vi "8.11.-Momentos Invariantes de Hu - Reconocimiento Patrones.vi"(7 "Normalización":bool, 9 "UMBRAL":dbl(knob) scale=0.0..255.0, 10 "CAPA DE COLOR":T1(ring), 11 "RUTA DE IMAGEN":path) -> (2 "Momentos Invariantes de Hu":dbl[](array[numeric]), 3 "IMAGEN BINARIZADA":picture)   [LabVIEW 2020]
panel:
  in  "Filtro Invertido":bool
  # "Visión Artificial - Momentos Invariantes de Hu\nDiego Cervantes Rodríguez\ndicer0.com"
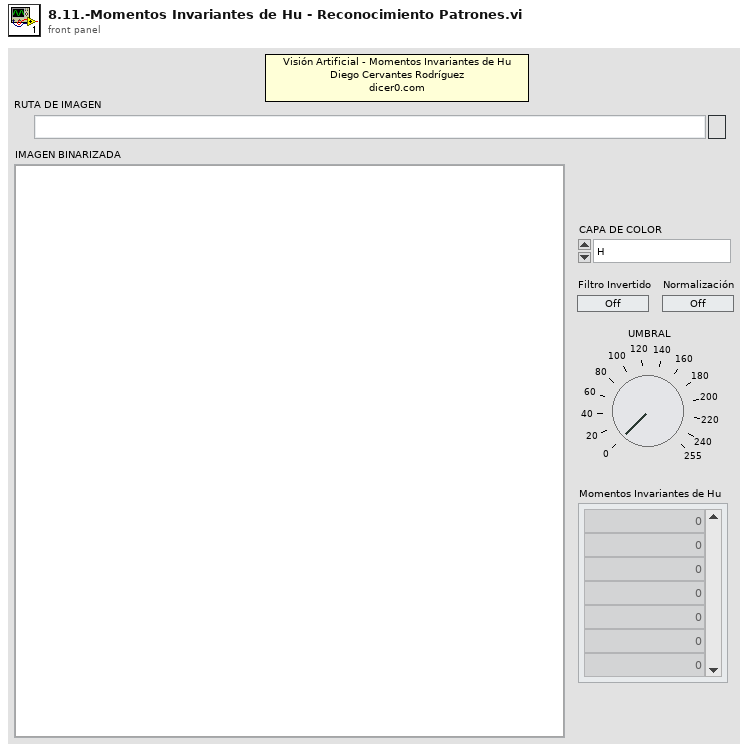
[diagram p1: front panel]
types:
  T1 = enum16{"H", "S", "V", "C", "M", "Y", "R", "G", "B", "RGB2GRAY MATLAB"}
  T2 = typedef "imagedata.ctl" = cluster{"image type":i32, "image depth":i32, "image":u8[], "mask":u8[], "colors":u32[], "Rectangle":cluster{"left":i16, "top":i16, "right":i16, "bottom":i16}}
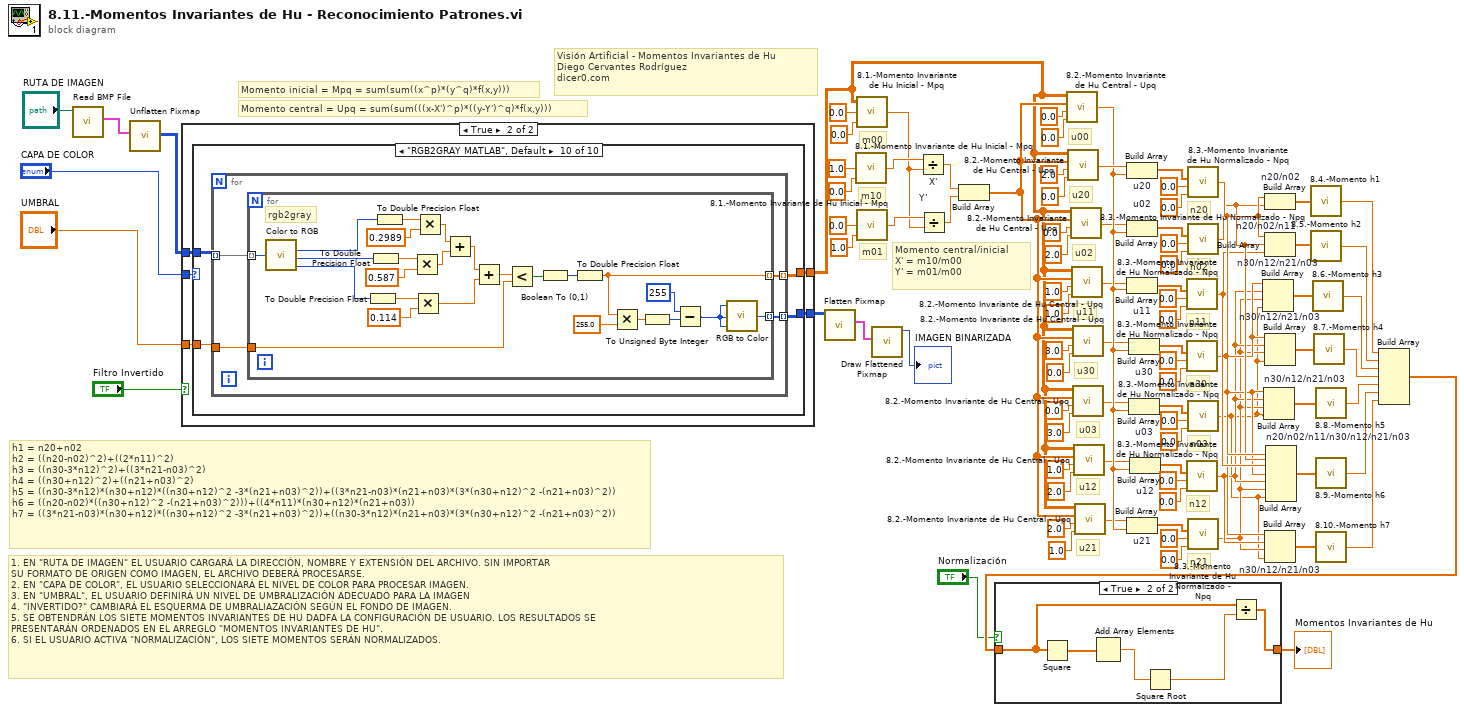
[diagram p0: block diagram]
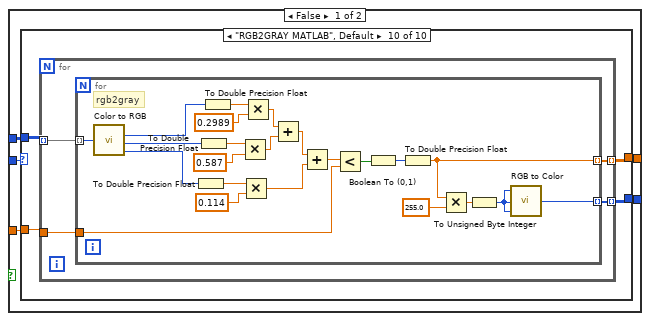
[diagram p2: hidden frame]
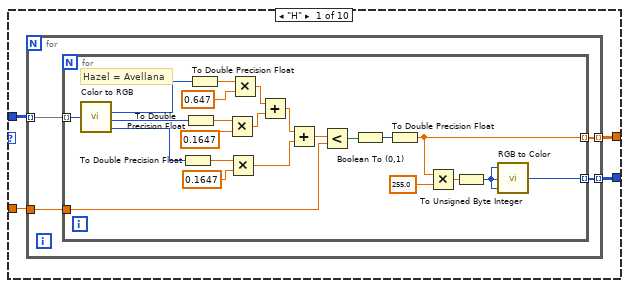
[diagram p3: hidden frame]
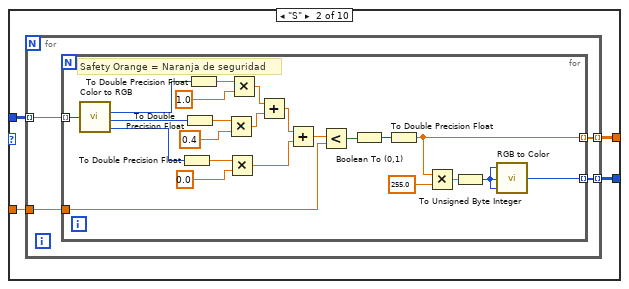
[diagram p4: hidden frame]
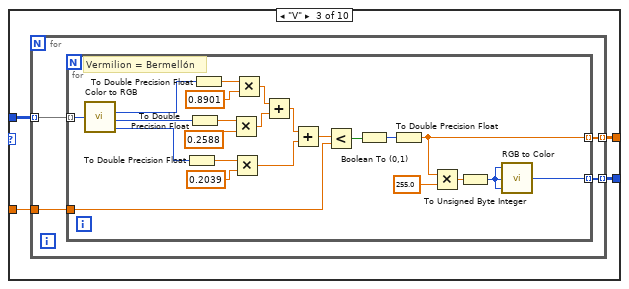
[diagram p5: hidden frame]
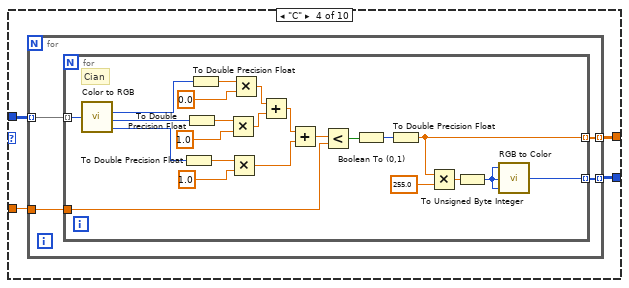
[diagram p6: hidden frame]
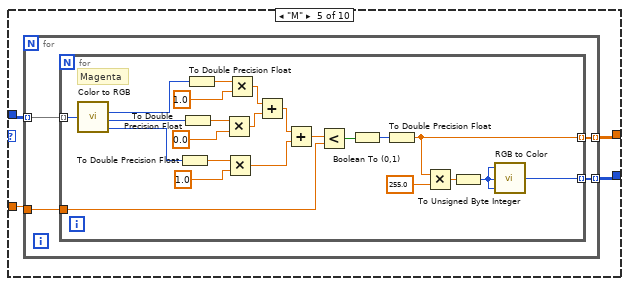
[diagram p7: hidden frame]
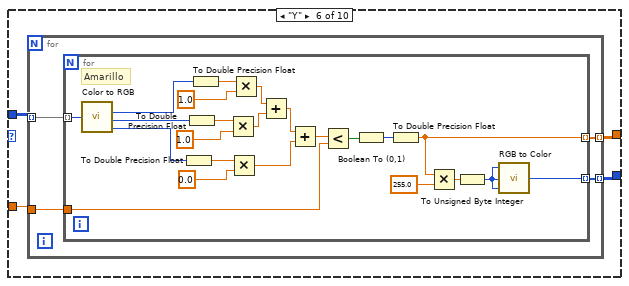
[diagram p8: hidden frame]
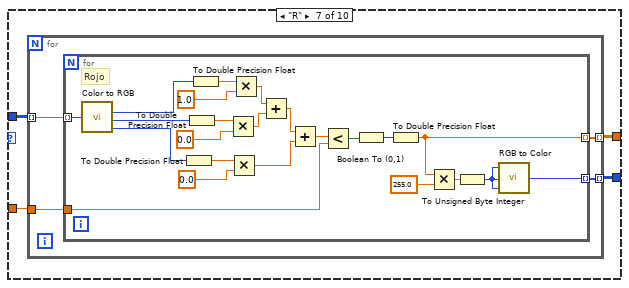
[diagram p9: hidden frame]
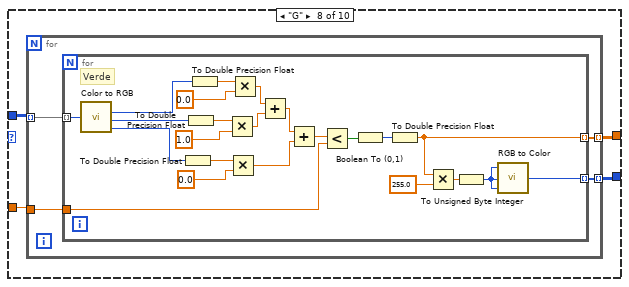
[diagram p10: hidden frame]
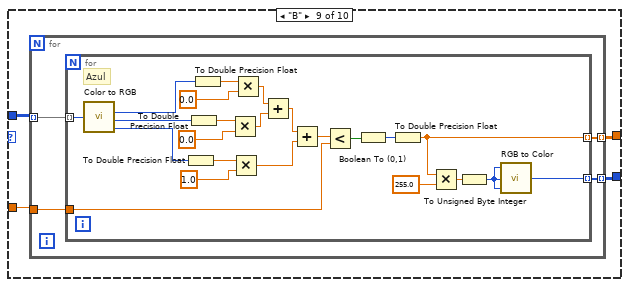
[diagram p11: hidden frame]
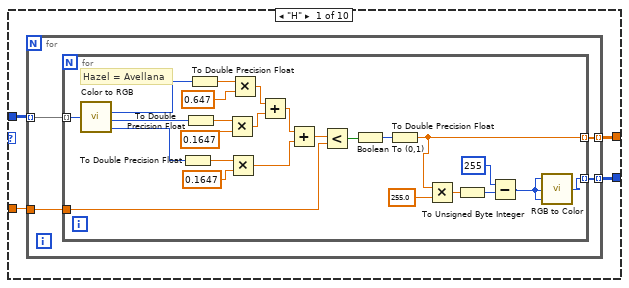
[diagram p12: hidden frame]
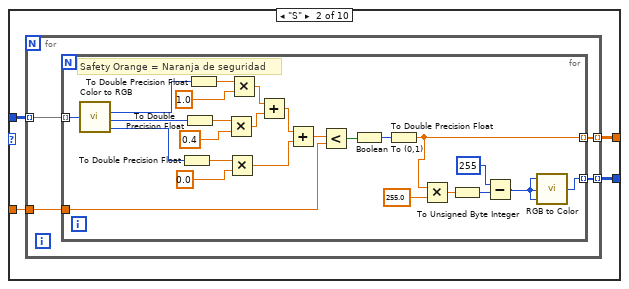
[diagram p13: hidden frame]
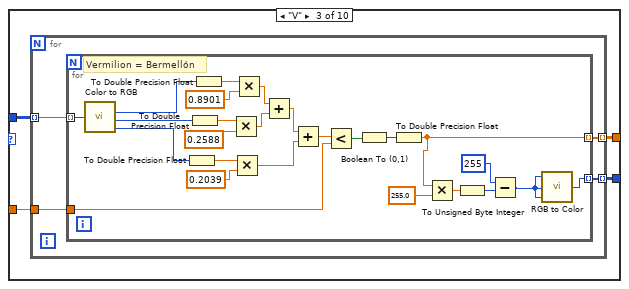
[diagram p14: hidden frame]
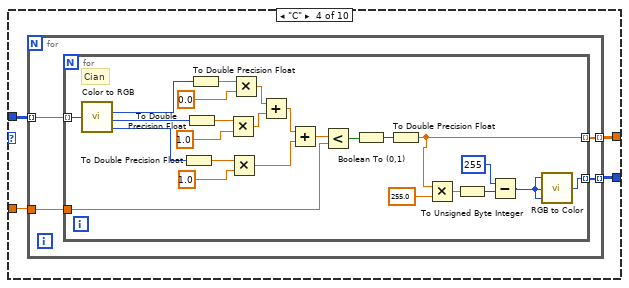
[diagram p15: hidden frame]
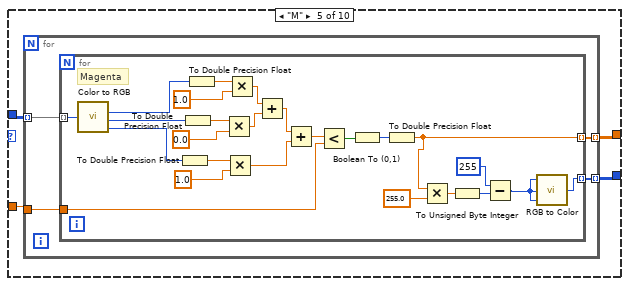
[diagram p16: hidden frame]
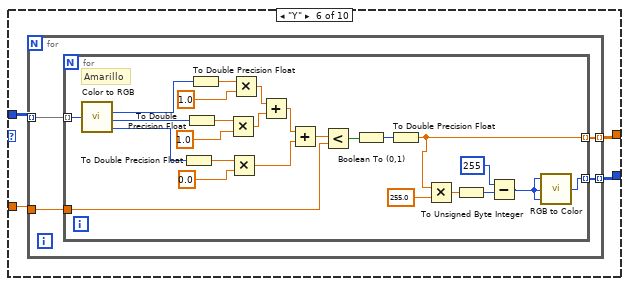
[diagram p17: hidden frame]
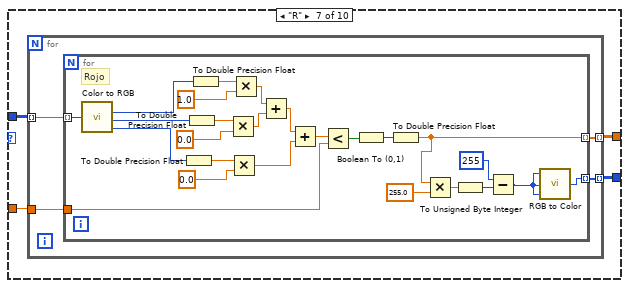
[diagram p18: hidden frame]
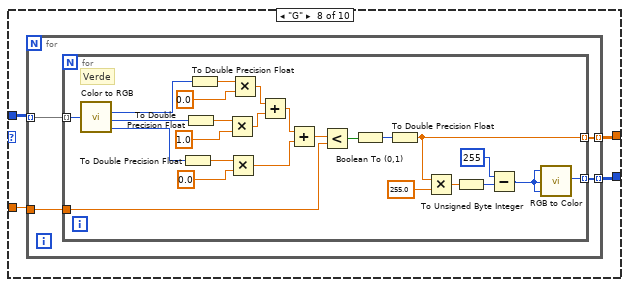
[diagram p19: hidden frame]
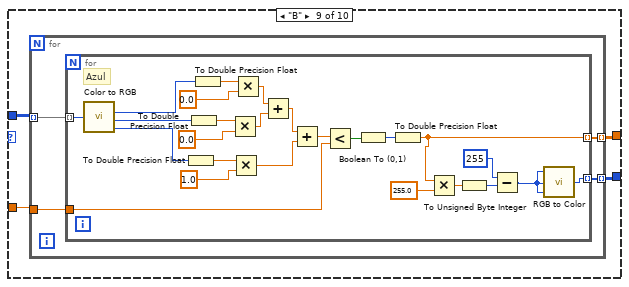
[diagram p20: hidden frame]
diagram:
  # "Visión Artificial - Momentos Invariantes de Hu\nDiego Cervantes Rodríguez\ndicer0.com"
  # "n21"
  # "n12"
  # "n03"
  # "n30"
  # "n11"
  # "n02"
  # "n20"
  # "u03"
  # "u21"
  # "u12"
  # "u30"
  # "u11"
  # "u02"
  # "Momento central = Upq = sum(sum(((x-X')^p)*((y-Y')^q)*f(x,y)))"
  # "Momento inicial = Mpq = sum(sum((x^p)*(y^q)*f(x,y)))"
  # "h1 = n20+n02\nh2 = ((n20-n02)^2)+((2*n11)^2)\nh3 = ((n30-3*n12)^2)+((3*n21-n03)^2)\nh4 = ((n30+n12)^2)+((n21+n03)^2)\nh5 = ((n30-3*n12)*(n30+n12)*((n30+n12)^2 -3*(n21+n03)^2))+((3*n21-n03)*(n21+n03)*(3*(n30+n12)^2 -(n21+n03)^2))\nh6 = ((n20-n02)*((n30+n12)^2 -(n21+n03)^2)))+((4*n11)*(n30+n12)*(n21+n03))\nh7 = ((3*n21-n03)*(n30+n12)*((n30+n12)^2 -3*(n21+n03)^2))+((n30-3*n12)*(n21+n03)*(3*(n30+n12)^2 -(n21+n03)^2))"
  # "u20"
  # "u00"
  # "Momento central/inicial\nX' = m10/m00 \nY' = m01/m00"
  # "m10"
  # "m01"
  # "m00"
  # "1. EN \"RUTA DE IMAGEN\" EL USUARIO CARGARÁ LA DIRECCIÓN, NOMBRE Y EXTENSIÓN DEL ARCHIVO. SIN IMPORTAR \nSU FORMATO DE ORIGEN COMO IMAGEN, EL ARCHIVO DEBERÁ PROCESARSE. \n2. EN \"CAPA DE COLOR\", EL USUARIO SELECCIONARÁ EL NIVEL DE COLOR PARA PROCESAR IMAGEN. \n3. EN \"UMBRAL\", EL USUARIO DEFINIRÁ UN NIVEL DE UMBRALIZACIÓN ADECUADO PARA LA IMAGEN \n4. \"INVERTIDO?\" CAMBIARÁ EL ESQUERMA DE UMBRALIAZACIÓN SEGÚN EL FONDO DE IMAGEN. \n5. SE OBTENDRÁN LOS SIETE MOMENTOS INVARIANTES DE HU DADFA LA CONFIGURACIÓN DE USUARIO. LOS RESULTADOS SE \nPRESENTARÁN ORDENADOS EN EL ARREGLO \"MOMENTOS INVARIANTES DE HU\".\n6. SI EL USUARIO ACTIVA \"NORMALIZACIÓN\", LOS SIETE MOMENTOS SERÁN NORMALIZADOS."
  n1 = call <vilib>:"Read BMP File.vi"("path to BMP file"="RUTA DE IMAGEN") -> ("image data"=w91:T2)  [unwired: 8 in, 2 out]
  n2 = call <vilib>:"Unflatten Pixmap.vi"("image data"=w91) -> ("24-bit pixmap"=w90:u32[][])  [unwired: 4 in, 6 out]
  n3 = case shown="True" "Filtro Invertido" {
    tunnel: w90 -> [w93 w411]
    tunnel: "UMBRAL" -> [w94 w410]
    tunnel: [w95 w409] -> w86
    tunnel: [w96 w408] -> w56
    tunnel: "CAPA DE COLOR" -> [w92 w407]
    frame False {
      n4 = case shown="\"RGB2GRAY MATLAB\", Default" w92 {
        tunnel: w93 -> [w100 w131 w162 w193 w224 w255 w286 w317 w347 w378]
        tunnel: w94 -> [w99 w130 w161 w192 w223 w254 w285 w316 w348 w379]
        tunnel: [w98 w129 w159 w191 w221 w252 w283 w315 w345 w377] -> w95
        tunnel: [w97 w128 w160 w190 w222 w253 w284 w314 w346 w376] -> w96
        frame "H" {
          n5 = for {
            tunnel: w100 -> [w104] mode=indexing
            tunnel: [w103] -> w97 mode=indexing
            tunnel: [w102] -> w98 mode=indexing
            tunnel: w99 -> [w101]
            n6 = for {
              tunnel: w104 -> [w127] mode=indexing
              tunnel: [w121] -> w103 mode=indexing
              tunnel: [w117] -> w102 mode=indexing
              tunnel: w101 -> [w110]
              # "Hazel = Avellana"
              n7 = call <vilib>:"Color to RGB.vi"("Color"=w127) -> ("R"=w116:u8, "G"=w114:u8, "B"=w112:u8)  [unwired: 1 out]
              n8 = To Double Precision Float(number=w112) -> (double precision float=w111:dbl)
              n9 = To Double Precision Float(number=w114) -> (double precision float=w113:dbl)
              n10 = To Double Precision Float(number=w116) -> (double precision float=w115:dbl)
              n11 = Multiply(x=w113, y=0.1647) -> (x*y=w107:dbl)
              n12 = Multiply(x=w111, y=0.1647) -> (x*y=w108:dbl)
              n13 = Multiply(x=w115, y=0.647) -> (x*y=w106:dbl)
              n14 = Add(x=w106, y=w107) -> (x+y=w109:dbl)
              n15 = Add(x=w109, y=w108) -> (x+y=w105:dbl)
              n16 = Less?(x=w105, y=w110) -> (x < y?=w123:bool)
              n17 = Boolean To (0,1)(Boolean=w123) -> (0, 1=w122:i16)
              n18 = To Double Precision Float(number=w122) -> (double precision float=w121:dbl)
              n19 = Multiply(x=w121, y=255.0) -> (x*y=w119:dbl)
              n20 = To Unsigned Byte Integer(number=w119) -> (unsigned 8bit integer=w118:u8)
              n21 = call <vilib>:"RGB to Color.vi"("B"=w118, "G"=w118, "R"=w118) -> ("Color"=w117:u32)
            }
          }
        }
        frame "S" {
          n22 = for {
            tunnel: w131 -> [w135] mode=indexing
            tunnel: [w134] -> w128 mode=indexing
            tunnel: [w133] -> w129 mode=indexing
            tunnel: w130 -> [w132]
            n23 = for {
              tunnel: w135 -> [w158] mode=indexing
              tunnel: [w152] -> w134 mode=indexing
              tunnel: [w148] -> w133 mode=indexing
              tunnel: w132 -> [w141]
              # "Safety Orange = Naranja de seguridad"
              n24 = call <vilib>:"Color to RGB.vi"("Color"=w158) -> ("R"=w147:u8, "G"=w145:u8, "B"=w143:u8)  [unwired: 1 out]
              n25 = To Double Precision Float(number=w143) -> (double precision float=w142:dbl)
              n26 = To Double Precision Float(number=w145) -> (double precision float=w144:dbl)
              n27 = To Double Precision Float(number=w147) -> (double precision float=w146:dbl)
              n28 = Multiply(x=w144, y=0.4) -> (x*y=w138:dbl)
              n29 = Multiply(x=w142, y=0.0) -> (x*y=w139:dbl)
              n30 = Multiply(x=w146, y=1.0) -> (x*y=w137:dbl)
              n31 = Add(x=w137, y=w138) -> (x+y=w140:dbl)
              n32 = Add(x=w140, y=w139) -> (x+y=w136:dbl)
              n33 = Less?(x=w136, y=w141) -> (x < y?=w154:bool)
              n34 = Boolean To (0,1)(Boolean=w154) -> (0, 1=w153:i16)
              n35 = To Double Precision Float(number=w153) -> (double precision float=w152:dbl)
              n36 = Multiply(x=w152, y=255.0) -> (x*y=w150:dbl)
              n37 = To Unsigned Byte Integer(number=w150) -> (unsigned 8bit integer=w149:u8)
              n38 = call <vilib>:"RGB to Color.vi"("B"=w149, "G"=w149, "R"=w149) -> ("Color"=w148:u32)
            }
          }
        }
        frame "V" {
          n39 = for {
            tunnel: w162 -> [w166] mode=indexing
            tunnel: [w165] -> w160 mode=indexing
            tunnel: [w164] -> w159 mode=indexing
            tunnel: w161 -> [w163]
            n40 = for {
              tunnel: w166 -> [w189] mode=indexing
              tunnel: [w183] -> w165 mode=indexing
              tunnel: [w179] -> w164 mode=indexing
              tunnel: w163 -> [w172]
              # "Vermilion = Bermellón"
              n41 = call <vilib>:"Color to RGB.vi"("Color"=w189) -> ("R"=w178:u8, "G"=w176:u8, "B"=w174:u8)  [unwired: 1 out]
              n42 = To Double Precision Float(number=w174) -> (double precision float=w173:dbl)
              n43 = To Double Precision Float(number=w176) -> (double precision float=w175:dbl)
              n44 = To Double Precision Float(number=w178) -> (double precision float=w177:dbl)
              n45 = Multiply(x=w175, y=0.2588) -> (x*y=w169:dbl)
              n46 = Multiply(x=w173, y=0.2039) -> (x*y=w170:dbl)
              n47 = Multiply(x=w177, y=0.8901) -> (x*y=w168:dbl)
              n48 = Add(x=w168, y=w169) -> (x+y=w171:dbl)
              n49 = Add(x=w171, y=w170) -> (x+y=w167:dbl)
              n50 = Less?(x=w167, y=w172) -> (x < y?=w185:bool)
              n51 = Boolean To (0,1)(Boolean=w185) -> (0, 1=w184:i16)
              n52 = To Double Precision Float(number=w184) -> (double precision float=w183:dbl)
              n53 = Multiply(x=w183, y=255.0) -> (x*y=w181:dbl)
              n54 = To Unsigned Byte Integer(number=w181) -> (unsigned 8bit integer=w180:u8)
              n55 = call <vilib>:"RGB to Color.vi"("B"=w180, "G"=w180, "R"=w180) -> ("Color"=w179:u32)
            }
          }
        }
        frame "C" {
          n56 = for {
            tunnel: w193 -> [w197] mode=indexing
            tunnel: [w196] -> w190 mode=indexing
            tunnel: [w195] -> w191 mode=indexing
            tunnel: w192 -> [w194]
            n57 = for {
              tunnel: w197 -> [w220] mode=indexing
              tunnel: [w214] -> w196 mode=indexing
              tunnel: [w210] -> w195 mode=indexing
              tunnel: w194 -> [w203]
              # "Cian"
              n58 = call <vilib>:"Color to RGB.vi"("Color"=w220) -> ("R"=w209:u8, "G"=w207:u8, "B"=w205:u8)  [unwired: 1 out]
              n59 = To Double Precision Float(number=w205) -> (double precision float=w204:dbl)
              n60 = To Double Precision Float(number=w207) -> (double precision float=w206:dbl)
              n61 = To Double Precision Float(number=w209) -> (double precision float=w208:dbl)
              n62 = Multiply(x=w206, y=1.0) -> (x*y=w200:dbl)
              n63 = Multiply(x=w204, y=1.0) -> (x*y=w201:dbl)
              n64 = Multiply(x=w208, y=0.0) -> (x*y=w199:dbl)
              n65 = Add(x=w199, y=w200) -> (x+y=w202:dbl)
              n66 = Add(x=w202, y=w201) -> (x+y=w198:dbl)
              n67 = Less?(x=w198, y=w203) -> (x < y?=w216:bool)
              n68 = Boolean To (0,1)(Boolean=w216) -> (0, 1=w215:i16)
              n69 = To Double Precision Float(number=w215) -> (double precision float=w214:dbl)
              n70 = Multiply(x=w214, y=255.0) -> (x*y=w212:dbl)
              n71 = To Unsigned Byte Integer(number=w212) -> (unsigned 8bit integer=w211:u8)
              n72 = call <vilib>:"RGB to Color.vi"("B"=w211, "G"=w211, "R"=w211) -> ("Color"=w210:u32)
            }
          }
        }
        frame "M" {
          n73 = for {
            tunnel: w224 -> [w228] mode=indexing
            tunnel: [w227] -> w222 mode=indexing
            tunnel: [w226] -> w221 mode=indexing
            tunnel: w223 -> [w225]
            n74 = for {
              tunnel: w228 -> [w251] mode=indexing
              tunnel: [w245] -> w227 mode=indexing
              tunnel: [w241] -> w226 mode=indexing
              tunnel: w225 -> [w234]
              # "Magenta"
              n75 = call <vilib>:"Color to RGB.vi"("Color"=w251) -> ("R"=w240:u8, "G"=w238:u8, "B"=w236:u8)  [unwired: 1 out]
              n76 = To Double Precision Float(number=w236) -> (double precision float=w235:dbl)
              n77 = To Double Precision Float(number=w238) -> (double precision float=w237:dbl)
              n78 = To Double Precision Float(number=w240) -> (double precision float=w239:dbl)
              n79 = Multiply(x=w237, y=0.0) -> (x*y=w231:dbl)
              n80 = Multiply(x=w235, y=1.0) -> (x*y=w232:dbl)
              n81 = Multiply(x=w239, y=1.0) -> (x*y=w230:dbl)
              n82 = Add(x=w230, y=w231) -> (x+y=w233:dbl)
              n83 = Add(x=w233, y=w232) -> (x+y=w229:dbl)
              n84 = Less?(x=w229, y=w234) -> (x < y?=w247:bool)
              n85 = Boolean To (0,1)(Boolean=w247) -> (0, 1=w246:i16)
              n86 = To Double Precision Float(number=w246) -> (double precision float=w245:dbl)
              n87 = Multiply(x=w245, y=255.0) -> (x*y=w243:dbl)
              n88 = To Unsigned Byte Integer(number=w243) -> (unsigned 8bit integer=w242:u8)
              n89 = call <vilib>:"RGB to Color.vi"("B"=w242, "G"=w242, "R"=w242) -> ("Color"=w241:u32)
            }
          }
        }
        frame "Y" {
          n90 = for {
            tunnel: w255 -> [w259] mode=indexing
            tunnel: [w258] -> w253 mode=indexing
            tunnel: [w257] -> w252 mode=indexing
            tunnel: w254 -> [w256]
            n91 = for {
              tunnel: w259 -> [w282] mode=indexing
              tunnel: [w276] -> w258 mode=indexing
              tunnel: [w272] -> w257 mode=indexing
              tunnel: w256 -> [w265]
              # "Amarillo"
              n92 = call <vilib>:"Color to RGB.vi"("Color"=w282) -> ("R"=w271:u8, "G"=w269:u8, "B"=w267:u8)  [unwired: 1 out]
              n93 = To Double Precision Float(number=w267) -> (double precision float=w266:dbl)
              n94 = To Double Precision Float(number=w269) -> (double precision float=w268:dbl)
              n95 = To Double Precision Float(number=w271) -> (double precision float=w270:dbl)
              n96 = Multiply(x=w268, y=1.0) -> (x*y=w262:dbl)
              n97 = Multiply(x=w266, y=0.0) -> (x*y=w263:dbl)
              n98 = Multiply(x=w270, y=1.0) -> (x*y=w261:dbl)
              n99 = Add(x=w261, y=w262) -> (x+y=w264:dbl)
              n100 = Add(x=w264, y=w263) -> (x+y=w260:dbl)
              n101 = Less?(x=w260, y=w265) -> (x < y?=w278:bool)
              n102 = Boolean To (0,1)(Boolean=w278) -> (0, 1=w277:i16)
              n103 = To Double Precision Float(number=w277) -> (double precision float=w276:dbl)
              n104 = Multiply(x=w276, y=255.0) -> (x*y=w274:dbl)
              n105 = To Unsigned Byte Integer(number=w274) -> (unsigned 8bit integer=w273:u8)
              n106 = call <vilib>:"RGB to Color.vi"("B"=w273, "G"=w273, "R"=w273) -> ("Color"=w272:u32)
            }
          }
        }
        frame "R" {
          n107 = for {
            tunnel: w286 -> [w290] mode=indexing
            tunnel: [w289] -> w284 mode=indexing
            tunnel: [w288] -> w283 mode=indexing
            tunnel: w285 -> [w287]
            n108 = for {
              tunnel: w290 -> [w313] mode=indexing
              tunnel: [w307] -> w289 mode=indexing
              tunnel: [w303] -> w288 mode=indexing
              tunnel: w287 -> [w296]
              # "Rojo"
              n109 = call <vilib>:"Color to RGB.vi"("Color"=w313) -> ("R"=w302:u8, "G"=w300:u8, "B"=w298:u8)  [unwired: 1 out]
              n110 = To Double Precision Float(number=w298) -> (double precision float=w297:dbl)
              n111 = To Double Precision Float(number=w300) -> (double precision float=w299:dbl)
              n112 = To Double Precision Float(number=w302) -> (double precision float=w301:dbl)
              n113 = Multiply(x=w299, y=0.0) -> (x*y=w293:dbl)
              n114 = Multiply(x=w297, y=0.0) -> (x*y=w294:dbl)
              n115 = Multiply(x=w301, y=1.0) -> (x*y=w292:dbl)
              n116 = Add(x=w292, y=w293) -> (x+y=w295:dbl)
              n117 = Add(x=w295, y=w294) -> (x+y=w291:dbl)
              n118 = Less?(x=w291, y=w296) -> (x < y?=w309:bool)
              n119 = Boolean To (0,1)(Boolean=w309) -> (0, 1=w308:i16)
              n120 = To Double Precision Float(number=w308) -> (double precision float=w307:dbl)
              n121 = Multiply(x=w307, y=255.0) -> (x*y=w305:dbl)
              n122 = To Unsigned Byte Integer(number=w305) -> (unsigned 8bit integer=w304:u8)
              n123 = call <vilib>:"RGB to Color.vi"("B"=w304, "G"=w304, "R"=w304) -> ("Color"=w303:u32)
            }
          }
        }
        frame "G" {
          n124 = for {
            tunnel: w317 -> [w321] mode=indexing
            tunnel: [w320] -> w314 mode=indexing
            tunnel: [w319] -> w315 mode=indexing
            tunnel: w316 -> [w318]
            n125 = for {
              tunnel: w321 -> [w344] mode=indexing
              tunnel: [w338] -> w320 mode=indexing
              tunnel: [w334] -> w319 mode=indexing
              tunnel: w318 -> [w327]
              # "Verde"
              n126 = call <vilib>:"Color to RGB.vi"("Color"=w344) -> ("R"=w333:u8, "G"=w331:u8, "B"=w329:u8)  [unwired: 1 out]
              n127 = To Double Precision Float(number=w329) -> (double precision float=w328:dbl)
              n128 = To Double Precision Float(number=w331) -> (double precision float=w330:dbl)
              n129 = To Double Precision Float(number=w333) -> (double precision float=w332:dbl)
              n130 = Multiply(x=w330, y=1.0) -> (x*y=w324:dbl)
              n131 = Multiply(x=w328, y=0.0) -> (x*y=w325:dbl)
              n132 = Multiply(x=w332, y=0.0) -> (x*y=w323:dbl)
              n133 = Add(x=w323, y=w324) -> (x+y=w326:dbl)
              n134 = Add(x=w326, y=w325) -> (x+y=w322:dbl)
              n135 = Less?(x=w322, y=w327) -> (x < y?=w340:bool)
              n136 = Boolean To (0,1)(Boolean=w340) -> (0, 1=w339:i16)
              n137 = To Double Precision Float(number=w339) -> (double precision float=w338:dbl)
              n138 = Multiply(x=w338, y=255.0) -> (x*y=w336:dbl)
              n139 = To Unsigned Byte Integer(number=w336) -> (unsigned 8bit integer=w335:u8)
              n140 = call <vilib>:"RGB to Color.vi"("B"=w335, "G"=w335, "R"=w335) -> ("Color"=w334:u32)
            }
          }
        }
        frame "B" {
          n141 = for {
            tunnel: w347 -> [w352] mode=indexing
            tunnel: [w351] -> w346 mode=indexing
            tunnel: [w350] -> w345 mode=indexing
            tunnel: w348 -> [w349]
            n142 = for {
              tunnel: w352 -> [w375] mode=indexing
              tunnel: [w369] -> w351 mode=indexing
              tunnel: [w365] -> w350 mode=indexing
              tunnel: w349 -> [w358]
              # "Azul"
              n143 = call <vilib>:"Color to RGB.vi"("Color"=w375) -> ("R"=w364:u8, "G"=w362:u8, "B"=w360:u8)  [unwired: 1 out]
              n144 = To Double Precision Float(number=w360) -> (double precision float=w359:dbl)
              n145 = To Double Precision Float(number=w362) -> (double precision float=w361:dbl)
              n146 = To Double Precision Float(number=w364) -> (double precision float=w363:dbl)
              n147 = Multiply(x=w361, y=0.0) -> (x*y=w355:dbl)
              n148 = Multiply(x=w359, y=1.0) -> (x*y=w356:dbl)
              n149 = Multiply(x=w363, y=0.0) -> (x*y=w354:dbl)
              n150 = Add(x=w354, y=w355) -> (x+y=w357:dbl)
              n151 = Add(x=w357, y=w356) -> (x+y=w353:dbl)
              n152 = Less?(x=w353, y=w358) -> (x < y?=w371:bool)
              n153 = Boolean To (0,1)(Boolean=w371) -> (0, 1=w370:i16)
              n154 = To Double Precision Float(number=w370) -> (double precision float=w369:dbl)
              n155 = Multiply(x=w369, y=255.0) -> (x*y=w367:dbl)
              n156 = To Unsigned Byte Integer(number=w367) -> (unsigned 8bit integer=w366:u8)
              n157 = call <vilib>:"RGB to Color.vi"("B"=w366, "G"=w366, "R"=w366) -> ("Color"=w365:u32)
            }
          }
        }
        frame "RGB2GRAY MATLAB", Default {
          n158 = for {
            tunnel: w378 -> [w383] mode=indexing
            tunnel: [w382] -> w376 mode=indexing
            tunnel: [w381] -> w377 mode=indexing
            tunnel: w379 -> [w380]
            n159 = for {
              tunnel: w383 -> [w406] mode=indexing
              tunnel: [w400] -> w382 mode=indexing
              tunnel: [w396] -> w381 mode=indexing
              tunnel: w380 -> [w389]
              # "rgb2gray"
              n160 = call <vilib>:"Color to RGB.vi"("Color"=w406) -> ("R"=w395:u8, "G"=w393:u8, "B"=w391:u8)  [unwired: 1 out]
              n161 = To Double Precision Float(number=w391) -> (double precision float=w390:dbl)
              n162 = To Double Precision Float(number=w393) -> (double precision float=w392:dbl)
              n163 = To Double Precision Float(number=w395) -> (double precision float=w394:dbl)
              n164 = Multiply(x=w392, y=0.587) -> (x*y=w386:dbl)
              n165 = Multiply(x=w390, y=0.114) -> (x*y=w387:dbl)
              n166 = Multiply(x=w394, y=0.2989) -> (x*y=w385:dbl)
              n167 = Add(x=w385, y=w386) -> (x+y=w388:dbl)
              n168 = Add(x=w388, y=w387) -> (x+y=w384:dbl)
              n169 = Less?(x=w384, y=w389) -> (x < y?=w402:bool)
              n170 = Boolean To (0,1)(Boolean=w402) -> (0, 1=w401:i16)
              n171 = To Double Precision Float(number=w401) -> (double precision float=w400:dbl)
              n172 = Multiply(x=w400, y=255.0) -> (x*y=w398:dbl)
              n173 = To Unsigned Byte Integer(number=w398) -> (unsigned 8bit integer=w397:u8)
              n174 = call <vilib>:"RGB to Color.vi"("B"=w397, "G"=w397, "R"=w397) -> ("Color"=w396:u32)
            }
          }
        }
      }
    }
    frame True {
      n175 = case shown="\"RGB2GRAY MATLAB\", Default" w407 {
        tunnel: w411 -> [w415 w448 w481 w514 w547 w580 w613 w646 w678 w711]
        tunnel: w410 -> [w414 w447 w480 w513 w546 w579 w612 w645 w679 w712]
        tunnel: [w413 w446 w478 w512 w544 w577 w610 w644 w676 w710] -> w409
        tunnel: [w412 w445 w479 w511 w545 w578 w611 w643 w677 w709] -> w408
        frame "H" {
          n176 = for {
            tunnel: w415 -> [w419] mode=indexing
            tunnel: [w418] -> w412 mode=indexing
            tunnel: [w417] -> w413 mode=indexing
            tunnel: w414 -> [w416]
            n177 = for {
              tunnel: w419 -> [w444] mode=indexing
              tunnel: [w421] -> w418 mode=indexing
              tunnel: [w420] -> w417 mode=indexing
              tunnel: w416 -> [w432]
              # "Hazel = Avellana"
              n178 = call <vilib>:"Color to RGB.vi"("Color"=w444) -> ("R"=w438:u8, "G"=w436:u8, "B"=w434:u8)  [unwired: 1 out]
              n179 = To Double Precision Float(number=w434) -> (double precision float=w433:dbl)
              n180 = To Double Precision Float(number=w436) -> (double precision float=w435:dbl)
              n181 = To Double Precision Float(number=w438) -> (double precision float=w437:dbl)
              n182 = Multiply(x=w435, y=0.1647) -> (x*y=w429:dbl)
              n183 = Multiply(x=w433, y=0.1647) -> (x*y=w430:dbl)
              n184 = Multiply(x=w437, y=0.647) -> (x*y=w428:dbl)
              n185 = Add(x=w428, y=w429) -> (x+y=w431:dbl)
              n186 = Add(x=w431, y=w430) -> (x+y=w427:dbl)
              n187 = Less?(x=w427, y=w432) -> (x < y?=w440:bool)
              n188 = Boolean To (0,1)(Boolean=w440) -> (0, 1=w439:i16)
              n189 = To Double Precision Float(number=w439) -> (double precision float=w421:dbl)
              n190 = Multiply(x=w421, y=255.0) -> (x*y=w425:dbl)
              n191 = To Unsigned Byte Integer(number=w425) -> (unsigned 8bit integer=w424:u8)
              n192 = Subtract(x=u8 255, y=w424) -> (x-y=w423:u8)
              n193 = call <vilib>:"RGB to Color.vi"("B"=w423, "G"=w423, "R"=w423) -> ("Color"=w420:u32)
            }
          }
        }
        frame "S" {
          n194 = for {
            tunnel: w448 -> [w452] mode=indexing
            tunnel: [w451] -> w445 mode=indexing
            tunnel: [w450] -> w446 mode=indexing
            tunnel: w447 -> [w449]
            n195 = for {
              tunnel: w452 -> [w477] mode=indexing
              tunnel: [w455] -> w451 mode=indexing
              tunnel: [w453] -> w450 mode=indexing
              tunnel: w449 -> [w465]
              # "Safety Orange = Naranja de seguridad"
              n196 = call <vilib>:"Color to RGB.vi"("Color"=w477) -> ("R"=w471:u8, "G"=w469:u8, "B"=w467:u8)  [unwired: 1 out]
              n197 = To Double Precision Float(number=w467) -> (double precision float=w466:dbl)
              n198 = To Double Precision Float(number=w469) -> (double precision float=w468:dbl)
              n199 = To Double Precision Float(number=w471) -> (double precision float=w470:dbl)
              n200 = Multiply(x=w468, y=0.4) -> (x*y=w462:dbl)
              n201 = Multiply(x=w466, y=0.0) -> (x*y=w463:dbl)
              n202 = Multiply(x=w470, y=1.0) -> (x*y=w461:dbl)
              n203 = Add(x=w461, y=w462) -> (x+y=w464:dbl)
              n204 = Add(x=w464, y=w463) -> (x+y=w460:dbl)
              n205 = Less?(x=w460, y=w465) -> (x < y?=w473:bool)
              n206 = Boolean To (0,1)(Boolean=w473) -> (0, 1=w472:i16)
              n207 = To Double Precision Float(number=w472) -> (double precision float=w455:dbl)
              n208 = Multiply(x=w455, y=255.0) -> (x*y=w458:dbl)
              n209 = To Unsigned Byte Integer(number=w458) -> (unsigned 8bit integer=w457:u8)
              n210 = Subtract(x=u8 255, y=w457) -> (x-y=w456:u8)
              n211 = call <vilib>:"RGB to Color.vi"("B"=w456, "G"=w456, "R"=w456) -> ("Color"=w453:u32)
            }
          }
        }
        frame "V" {
          n212 = for {
            tunnel: w481 -> [w485] mode=indexing
            tunnel: [w484] -> w479 mode=indexing
            tunnel: [w483] -> w478 mode=indexing
            tunnel: w480 -> [w482]
            n213 = for {
              tunnel: w485 -> [w510] mode=indexing
              tunnel: [w488] -> w484 mode=indexing
              tunnel: [w487] -> w483 mode=indexing
              tunnel: w482 -> [w498]
              # "Vermilion = Bermellón"
              n214 = call <vilib>:"Color to RGB.vi"("Color"=w510) -> ("R"=w504:u8, "G"=w502:u8, "B"=w500:u8)  [unwired: 1 out]
              n215 = To Double Precision Float(number=w500) -> (double precision float=w499:dbl)
              n216 = To Double Precision Float(number=w502) -> (double precision float=w501:dbl)
              n217 = To Double Precision Float(number=w504) -> (double precision float=w503:dbl)
              n218 = Multiply(x=w501, y=0.2588) -> (x*y=w495:dbl)
              n219 = Multiply(x=w499, y=0.2039) -> (x*y=w496:dbl)
              n220 = Multiply(x=w503, y=0.8901) -> (x*y=w494:dbl)
              n221 = Add(x=w494, y=w495) -> (x+y=w497:dbl)
              n222 = Add(x=w497, y=w496) -> (x+y=w493:dbl)
              n223 = Less?(x=w493, y=w498) -> (x < y?=w506:bool)
              n224 = Boolean To (0,1)(Boolean=w506) -> (0, 1=w505:i16)
              n225 = To Double Precision Float(number=w505) -> (double precision float=w488:dbl)
              n226 = Multiply(x=w488, y=255.0) -> (x*y=w491:dbl)
              n227 = To Unsigned Byte Integer(number=w491) -> (unsigned 8bit integer=w490:u8)
              n228 = Subtract(x=u8 255, y=w490) -> (x-y=w489:u8)
              n229 = call <vilib>:"RGB to Color.vi"("B"=w489, "G"=w489, "R"=w489) -> ("Color"=w487:u32)
            }
          }
        }
        frame "C" {
          n230 = for {
            tunnel: w514 -> [w518] mode=indexing
            tunnel: [w517] -> w511 mode=indexing
            tunnel: [w516] -> w512 mode=indexing
            tunnel: w513 -> [w515]
            n231 = for {
              tunnel: w518 -> [w543] mode=indexing
              tunnel: [w521] -> w517 mode=indexing
              tunnel: [w520] -> w516 mode=indexing
              tunnel: w515 -> [w531]
              # "Cian"
              n232 = call <vilib>:"Color to RGB.vi"("Color"=w543) -> ("R"=w537:u8, "G"=w535:u8, "B"=w533:u8)  [unwired: 1 out]
              n233 = To Double Precision Float(number=w533) -> (double precision float=w532:dbl)
              n234 = To Double Precision Float(number=w535) -> (double precision float=w534:dbl)
              n235 = To Double Precision Float(number=w537) -> (double precision float=w536:dbl)
              n236 = Multiply(x=w534, y=1.0) -> (x*y=w528:dbl)
              n237 = Multiply(x=w532, y=1.0) -> (x*y=w529:dbl)
              n238 = Multiply(x=w536, y=0.0) -> (x*y=w527:dbl)
              n239 = Add(x=w527, y=w528) -> (x+y=w530:dbl)
              n240 = Add(x=w530, y=w529) -> (x+y=w526:dbl)
              n241 = Less?(x=w526, y=w531) -> (x < y?=w539:bool)
              n242 = Boolean To (0,1)(Boolean=w539) -> (0, 1=w538:i16)
              n243 = To Double Precision Float(number=w538) -> (double precision float=w521:dbl)
              n244 = Multiply(x=w521, y=255.0) -> (x*y=w524:dbl)
              n245 = To Unsigned Byte Integer(number=w524) -> (unsigned 8bit integer=w523:u8)
              n246 = Subtract(x=u8 255, y=w523) -> (x-y=w522:u8)
              n247 = call <vilib>:"RGB to Color.vi"("B"=w522, "G"=w522, "R"=w522) -> ("Color"=w520:u32)
            }
          }
        }
        frame "M" {
          n248 = for {
            tunnel: w547 -> [w551] mode=indexing
            tunnel: [w550] -> w545 mode=indexing
            tunnel: [w549] -> w544 mode=indexing
            tunnel: w546 -> [w548]
            n249 = for {
              tunnel: w551 -> [w576] mode=indexing
              tunnel: [w554] -> w550 mode=indexing
              tunnel: [w553] -> w549 mode=indexing
              tunnel: w548 -> [w564]
              # "Magenta"
              n250 = call <vilib>:"Color to RGB.vi"("Color"=w576) -> ("R"=w570:u8, "G"=w568:u8, "B"=w566:u8)  [unwired: 1 out]
              n251 = To Double Precision Float(number=w566) -> (double precision float=w565:dbl)
              n252 = To Double Precision Float(number=w568) -> (double precision float=w567:dbl)
              n253 = To Double Precision Float(number=w570) -> (double precision float=w569:dbl)
              n254 = Multiply(x=w567, y=0.0) -> (x*y=w561:dbl)
              n255 = Multiply(x=w565, y=1.0) -> (x*y=w562:dbl)
              n256 = Multiply(x=w569, y=1.0) -> (x*y=w560:dbl)
              n257 = Add(x=w560, y=w561) -> (x+y=w563:dbl)
              n258 = Add(x=w563, y=w562) -> (x+y=w559:dbl)
              n259 = Less?(x=w559, y=w564) -> (x < y?=w572:bool)
              n260 = Boolean To (0,1)(Boolean=w572) -> (0, 1=w571:i16)
              n261 = To Double Precision Float(number=w571) -> (double precision float=w554:dbl)
              n262 = Multiply(x=w554, y=255.0) -> (x*y=w557:dbl)
              n263 = To Unsigned Byte Integer(number=w557) -> (unsigned 8bit integer=w556:u8)
              n264 = Subtract(x=u8 255, y=w556) -> (x-y=w555:u8)
              n265 = call <vilib>:"RGB to Color.vi"("B"=w555, "G"=w555, "R"=w555) -> ("Color"=w553:u32)
            }
          }
        }
        frame "Y" {
          n266 = for {
            tunnel: w580 -> [w584] mode=indexing
            tunnel: [w583] -> w578 mode=indexing
            tunnel: [w582] -> w577 mode=indexing
            tunnel: w579 -> [w581]
            n267 = for {
              tunnel: w584 -> [w609] mode=indexing
              tunnel: [w587] -> w583 mode=indexing
              tunnel: [w586] -> w582 mode=indexing
              tunnel: w581 -> [w597]
              # "Amarillo"
              n268 = call <vilib>:"Color to RGB.vi"("Color"=w609) -> ("R"=w603:u8, "G"=w601:u8, "B"=w599:u8)  [unwired: 1 out]
              n269 = To Double Precision Float(number=w599) -> (double precision float=w598:dbl)
              n270 = To Double Precision Float(number=w601) -> (double precision float=w600:dbl)
              n271 = To Double Precision Float(number=w603) -> (double precision float=w602:dbl)
              n272 = Multiply(x=w600, y=1.0) -> (x*y=w594:dbl)
              n273 = Multiply(x=w598, y=0.0) -> (x*y=w595:dbl)
              n274 = Multiply(x=w602, y=1.0) -> (x*y=w593:dbl)
              n275 = Add(x=w593, y=w594) -> (x+y=w596:dbl)
              n276 = Add(x=w596, y=w595) -> (x+y=w592:dbl)
              n277 = Less?(x=w592, y=w597) -> (x < y?=w605:bool)
              n278 = Boolean To (0,1)(Boolean=w605) -> (0, 1=w604:i16)
              n279 = To Double Precision Float(number=w604) -> (double precision float=w587:dbl)
              n280 = Multiply(x=w587, y=255.0) -> (x*y=w590:dbl)
              n281 = To Unsigned Byte Integer(number=w590) -> (unsigned 8bit integer=w589:u8)
              n282 = Subtract(x=u8 255, y=w589) -> (x-y=w588:u8)
              n283 = call <vilib>:"RGB to Color.vi"("B"=w588, "G"=w588, "R"=w588) -> ("Color"=w586:u32)
            }
          }
        }
        frame "R" {
          n284 = for {
            tunnel: w613 -> [w617] mode=indexing
            tunnel: [w616] -> w611 mode=indexing
            tunnel: [w615] -> w610 mode=indexing
            tunnel: w612 -> [w614]
            n285 = for {
              tunnel: w617 -> [w642] mode=indexing
              tunnel: [w619] -> w616 mode=indexing
              tunnel: [w618] -> w615 mode=indexing
              tunnel: w614 -> [w630]
              # "Rojo"
              n286 = call <vilib>:"Color to RGB.vi"("Color"=w642) -> ("R"=w636:u8, "G"=w634:u8, "B"=w632:u8)  [unwired: 1 out]
              n287 = To Double Precision Float(number=w632) -> (double precision float=w631:dbl)
              n288 = To Double Precision Float(number=w634) -> (double precision float=w633:dbl)
              n289 = To Double Precision Float(number=w636) -> (double precision float=w635:dbl)
              n290 = Multiply(x=w633, y=0.0) -> (x*y=w627:dbl)
              n291 = Multiply(x=w631, y=0.0) -> (x*y=w628:dbl)
              n292 = Multiply(x=w635, y=1.0) -> (x*y=w626:dbl)
              n293 = Add(x=w626, y=w627) -> (x+y=w629:dbl)
              n294 = Add(x=w629, y=w628) -> (x+y=w625:dbl)
              n295 = Less?(x=w625, y=w630) -> (x < y?=w638:bool)
              n296 = Boolean To (0,1)(Boolean=w638) -> (0, 1=w637:i16)
              n297 = To Double Precision Float(number=w637) -> (double precision float=w619:dbl)
              n298 = Multiply(x=w619, y=255.0) -> (x*y=w623:dbl)
              n299 = To Unsigned Byte Integer(number=w623) -> (unsigned 8bit integer=w622:u8)
              n300 = Subtract(x=u8 255, y=w622) -> (x-y=w621:u8)
              n301 = call <vilib>:"RGB to Color.vi"("B"=w621, "G"=w621, "R"=w621) -> ("Color"=w618:u32)
            }
          }
        }
        frame "G" {
          n302 = for {
            tunnel: w646 -> [w650] mode=indexing
            tunnel: [w649] -> w643 mode=indexing
            tunnel: [w648] -> w644 mode=indexing
            tunnel: w645 -> [w647]
            n303 = for {
              tunnel: w650 -> [w675] mode=indexing
              tunnel: [w653] -> w649 mode=indexing
              tunnel: [w652] -> w648 mode=indexing
              tunnel: w647 -> [w663]
              # "Verde"
              n304 = call <vilib>:"Color to RGB.vi"("Color"=w675) -> ("R"=w669:u8, "G"=w667:u8, "B"=w665:u8)  [unwired: 1 out]
              n305 = To Double Precision Float(number=w665) -> (double precision float=w664:dbl)
              n306 = To Double Precision Float(number=w667) -> (double precision float=w666:dbl)
              n307 = To Double Precision Float(number=w669) -> (double precision float=w668:dbl)
              n308 = Multiply(x=w666, y=1.0) -> (x*y=w660:dbl)
              n309 = Multiply(x=w664, y=0.0) -> (x*y=w661:dbl)
              n310 = Multiply(x=w668, y=0.0) -> (x*y=w659:dbl)
              n311 = Add(x=w659, y=w660) -> (x+y=w662:dbl)
              n312 = Add(x=w662, y=w661) -> (x+y=w658:dbl)
              n313 = Less?(x=w658, y=w663) -> (x < y?=w671:bool)
              n314 = Boolean To (0,1)(Boolean=w671) -> (0, 1=w670:i16)
              n315 = To Double Precision Float(number=w670) -> (double precision float=w653:dbl)
              n316 = Multiply(x=w653, y=255.0) -> (x*y=w656:dbl)
              n317 = To Unsigned Byte Integer(number=w656) -> (unsigned 8bit integer=w655:u8)
              n318 = Subtract(x=u8 255, y=w655) -> (x-y=w654:u8)
              n319 = call <vilib>:"RGB to Color.vi"("B"=w654, "G"=w654, "R"=w654) -> ("Color"=w652:u32)
            }
          }
        }
        frame "B" {
          n320 = for {
            tunnel: w678 -> [w683] mode=indexing
            tunnel: [w682] -> w677 mode=indexing
            tunnel: [w681] -> w676 mode=indexing
            tunnel: w679 -> [w680]
            n321 = for {
              tunnel: w683 -> [w708] mode=indexing
              tunnel: [w685] -> w682 mode=indexing
              tunnel: [w686] -> w681 mode=indexing
              tunnel: w680 -> [w696]
              # "Azul"
              n322 = call <vilib>:"Color to RGB.vi"("Color"=w708) -> ("R"=w702:u8, "G"=w700:u8, "B"=w698:u8)  [unwired: 1 out]
              n323 = To Double Precision Float(number=w698) -> (double precision float=w697:dbl)
              n324 = To Double Precision Float(number=w700) -> (double precision float=w699:dbl)
              n325 = To Double Precision Float(number=w702) -> (double precision float=w701:dbl)
              n326 = Multiply(x=w699, y=0.0) -> (x*y=w693:dbl)
              n327 = Multiply(x=w697, y=1.0) -> (x*y=w694:dbl)
              n328 = Multiply(x=w701, y=0.0) -> (x*y=w692:dbl)
              n329 = Add(x=w692, y=w693) -> (x+y=w695:dbl)
              n330 = Add(x=w695, y=w694) -> (x+y=w691:dbl)
              n331 = Less?(x=w691, y=w696) -> (x < y?=w704:bool)
              n332 = Boolean To (0,1)(Boolean=w704) -> (0, 1=w703:i16)
              n333 = To Double Precision Float(number=w703) -> (double precision float=w685:dbl)
              n334 = Multiply(x=w685, y=255.0) -> (x*y=w689:dbl)
              n335 = To Unsigned Byte Integer(number=w689) -> (unsigned 8bit integer=w688:u8)
              n336 = Subtract(x=u8 255, y=w688) -> (x-y=w687:u8)
              n337 = call <vilib>:"RGB to Color.vi"("B"=w687, "G"=w687, "R"=w687) -> ("Color"=w686:u32)
            }
          }
        }
        frame "RGB2GRAY MATLAB", Default {
          n338 = for {
            tunnel: w711 -> [w716] mode=indexing
            tunnel: [w715] -> w709 mode=indexing
            tunnel: [w714] -> w710 mode=indexing
            tunnel: w712 -> [w713]
            n339 = for {
              tunnel: w716 -> [w741] mode=indexing
              tunnel: [w735] -> w715 mode=indexing
              tunnel: [w732] -> w714 mode=indexing
              tunnel: w713 -> [w725]
              # "rgb2gray"
              n340 = call <vilib>:"Color to RGB.vi"("Color"=w741) -> ("R"=w731:u8, "G"=w729:u8, "B"=w727:u8)  [unwired: 1 out]
              n341 = To Double Precision Float(number=w727) -> (double precision float=w726:dbl)
              n342 = To Double Precision Float(number=w729) -> (double precision float=w728:dbl)
              n343 = To Double Precision Float(number=w731) -> (double precision float=w730:dbl)
              n344 = Multiply(x=w728, y=0.587) -> (x*y=w722:dbl)
              n345 = Multiply(x=w726, y=0.114) -> (x*y=w723:dbl)
              n346 = Multiply(x=w730, y=0.2989) -> (x*y=w721:dbl)
              n347 = Add(x=w721, y=w722) -> (x+y=w724:dbl)
              n348 = Add(x=w724, y=w723) -> (x+y=w720:dbl)
              n349 = Less?(x=w720, y=w725) -> (x < y?=w737:bool)
              n350 = Boolean To (0,1)(Boolean=w737) -> (0, 1=w736:i16)
              n351 = To Double Precision Float(number=w736) -> (double precision float=w735:dbl)
              n352 = Multiply(x=w735, y=255.0) -> (x*y=w733:dbl)
              n353 = To Unsigned Byte Integer(number=w733) -> (unsigned 8bit integer=w718:u8)
              n354 = Subtract(x=u8 255, y=w718) -> (x-y=w717:u8)
              n355 = call <vilib>:"RGB to Color.vi"("B"=w717, "G"=w717, "R"=w717) -> ("Color"=w732:u32)
            }
          }
        }
      }
    }
  }
  n356 = call <vilib>:"Flatten Pixmap.vi"("24-bit pixmap"=w86) -> ("image data"=w87:T2)  [unwired: 10 in]
  n357 = call "8.1.-Momento Invariante de Hu Inicial - Mpq.vi"("q"=0.0, "p"=1.0) -> ("Mpq"=w78:dbl)  [unwired: 1 in]
  n358 = call "8.1.-Momento Invariante de Hu Inicial - Mpq.vi"("q"=0.0, "p"=0.0, "f(x,y)"=w56) -> ("Mpq"=w76:dbl)
  n359 = call "8.1.-Momento Invariante de Hu Inicial - Mpq.vi"("q"=1.0, "p"=0.0) -> ("Mpq"=w77:dbl)  [unwired: 1 in]
  n360 = call <vilib>:"Draw Flattened Pixmap.vi"("image data"=w87) -> ("new picture"=→"IMAGEN BINARIZADA":picture)  [unwired: 8 in]
  n361 = Divide "X'"(x=w78, y=w76) -> (x/y=w75:dbl)
  n362 = Divide "Y'"(x=w77, y=w76) -> (x/y=w74:dbl)
  n363 = Build Array "Build Array"(w75, w74) -> (w57:dbl[])
  n364 = call "8.2.-Momento Invariante de Hu Central - Upq.vi"("q"=0.0, "p"=0.0, "X' Y'"=w57, "f(x,y)"=w56) -> ("Upq"=w54:dbl)
  n365 = call "8.2.-Momento Invariante de Hu Central - Upq.vi"("q"=0.0, "p"=2.0, "X' Y'"=w57, "f(x,y)"=w56) -> ("Upq"=w55:dbl)
  n366 = call "8.2.-Momento Invariante de Hu Central - Upq.vi"("q"=2.0, "p"=0.0, "X' Y'"=w57, "f(x,y)"=w56) -> ("Upq"=w53:dbl)
  n367 = call "8.2.-Momento Invariante de Hu Central - Upq.vi"("q"=1.0, "p"=1.0, "X' Y'"=w57, "f(x,y)"=w56) -> ("Upq"=w52:dbl)
  n368 = call "8.2.-Momento Invariante de Hu Central - Upq.vi"("q"=0.0, "p"=3.0, "X' Y'"=w57, "f(x,y)"=w56) -> ("Upq"=w51:dbl)
  n369 = call "8.2.-Momento Invariante de Hu Central - Upq.vi"("q"=3.0, "p"=0.0, "X' Y'"=w57, "f(x,y)"=w56) -> ("Upq"=w50:dbl)
  n370 = call "8.2.-Momento Invariante de Hu Central - Upq.vi"("q"=2.0, "p"=1.0, "X' Y'"=w57, "f(x,y)"=w56) -> ("Upq"=w49:dbl)
  n371 = call "8.2.-Momento Invariante de Hu Central - Upq.vi"("q"=1.0, "p"=2.0, "X' Y'"=w57, "f(x,y)"=w56) -> ("Upq"=w48:dbl)
  n372 = Build Array "u20"(w55, w54) -> (w45:dbl[])
  n373 = Build Array "u02"(w53, w54) -> (w27:dbl[])
  n374 = Build Array "u11"(w52, w54) -> (w28:dbl[])
  n375 = Build Array "u21"(w48, w54) -> (w32:dbl[])
  n376 = Build Array "u30"(w51, w54) -> (w29:dbl[])
  n377 = Build Array "u03"(w50, w54) -> (w30:dbl[])
  n378 = Build Array "u12"(w49, w54) -> (w31:dbl[])
  n379 = call "8.3.-Momento Invariante de Hu Normalizado - Npq.vi"("q"=0.0, "p"=0.0, "Upq/u00"=w28) -> ("Npq"=w24:dbl)  [unwired: 1 in]
  n380 = call "8.3.-Momento Invariante de Hu Normalizado - Npq.vi"("q"=0.0, "p"=0.0, "Upq/u00"=w29) -> ("Npq"=w23:dbl)  [unwired: 1 in]
  n381 = call "8.3.-Momento Invariante de Hu Normalizado - Npq.vi"("q"=0.0, "p"=0.0, "Upq/u00"=w31) -> ("Npq"=w22:dbl)  [unwired: 1 in]
  n382 = call "8.3.-Momento Invariante de Hu Normalizado - Npq.vi"("q"=0.0, "p"=0.0, "Upq/u00"=w45) -> ("Npq"=w26:dbl)  [unwired: 1 in]
  n383 = call "8.3.-Momento Invariante de Hu Normalizado - Npq.vi"("q"=0.0, "p"=0.0, "Upq/u00"=w27) -> ("Npq"=w25:dbl)  [unwired: 1 in]
  n384 = call "8.3.-Momento Invariante de Hu Normalizado - Npq.vi"("q"=0.0, "p"=0.0, "Upq/u00"=w30) -> ("Npq"=w20:dbl)  [unwired: 1 in]
  n385 = call "8.3.-Momento Invariante de Hu Normalizado - Npq.vi"("q"=0.0, "p"=0.0, "Upq/u00"=w32) -> ("Npq"=w21:dbl)  [unwired: 1 in]
  n386 = Build Array "n30/n12/n21/n03"(w23, w22, w21, w20) -> (w17:dbl[])
  n387 = Build Array "n30/n12/n21/n03"(w23, w22, w21, w20) -> (w15:dbl[])
  n388 = Build Array "n20/n02"(w26, w25) -> (w19:dbl[])
  n389 = Build Array "n20/n02/n11"(w26, w25, w24) -> (w18:dbl[])
  n390 = Build Array "n30/n12/n21/n03"(w23, w22, w21, w20) -> (w16:dbl[])
  n391 = Build Array "n30/n12/n21/n03"(w23, w22, w21, w20) -> (w13:dbl[])
  n392 = Build Array "n20/n02/n11/n30/n12/n21/n03"(w26, w25, w24, w23, w22, w21, w20) -> (w14:dbl[])
  n393 = call "8.4.-Momento h1.vi"("n20/n02"=w19) -> ("M1"=w12:dbl)
  n394 = call "8.5.-Momento h2.vi"("n20/n02/n11"=w18) -> ("M2"=w11:dbl)
  n395 = call "8.6.-Momento h3.vi"("n30/n12/n21/n03"=w17) -> ("M3"=w10:dbl)
  n396 = call "8.7.-Momento h4.vi"("n30/n12/n21/n03"=w16) -> ("M4"=w9:dbl)
  n397 = call "8.8.-Momento h5.vi"("n30/n12/n21/n03"=w15) -> ("M5"=w8:dbl)
  n398 = call "8.9.-Momento h6.vi"("n20/n02/n11/n30/n12/n21/n03"=w14) -> ("M6"=w7:dbl)
  n399 = call "8.10.-Momento h7.vi"("n30/n12/n21/n03"=w13) -> ("M7"=w6:dbl)
  n400 = Build Array "Build Array"(w12, w11, w10, w9, w8, w7, w6) -> (w3:dbl[])
  n401 = case shown="True" "Normalización" {
    tunnel: [w742 w743] -> w4
    tunnel: w3 -> [w742 w744]
    frame False {
    }
    frame True {
      n402 = Square(x=w744) -> (x^2=w747:dbl[])
      n403 = Add Array Elements(numeric array=w747) -> (sum=w746:dbl)
      n404 = Square Root(x=w746) -> (sqrt(x)=w745:dbl)
      n405 = Divide(x=w744, y=w745) -> (x/y=w743:dbl[])
    }
  }
  "Momentos Invariantes de Hu" <- w4
